vi "Init Plugin.vi"(8 "error in (no error)":errorcluster, 11 "RequestRestUI in":refnum<class "RequestRestUI.lvclass">) -> (0 "error out":errorcluster, 3 "RequestRestUI out":refnum<class "RequestRestUI.lvclass">)   [LabVIEW 2015]
uses:
  Plugin/Plugin.lvclass
  DatabaseManagement/Database.lvclass
  RequestRestUI.lvclass
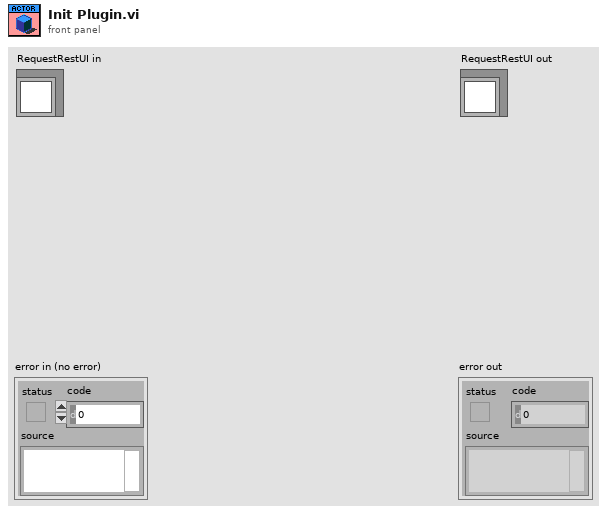
[diagram p1: front panel]
types:
  T1 = typedef "NI_Database_API.lvlib/DB Tools Column Info.ctl" = cluster{"column name":string, "data type":T2, "size":i32, "allow null?":bool}
  T2 = typedef "NI_Database_API.lvlib/DB Tools DataTypes.ctl" = enum16{"String", "Long (I32)", "Single (SGL)", "Double (DBL)", "Date/Time", "Binary"}
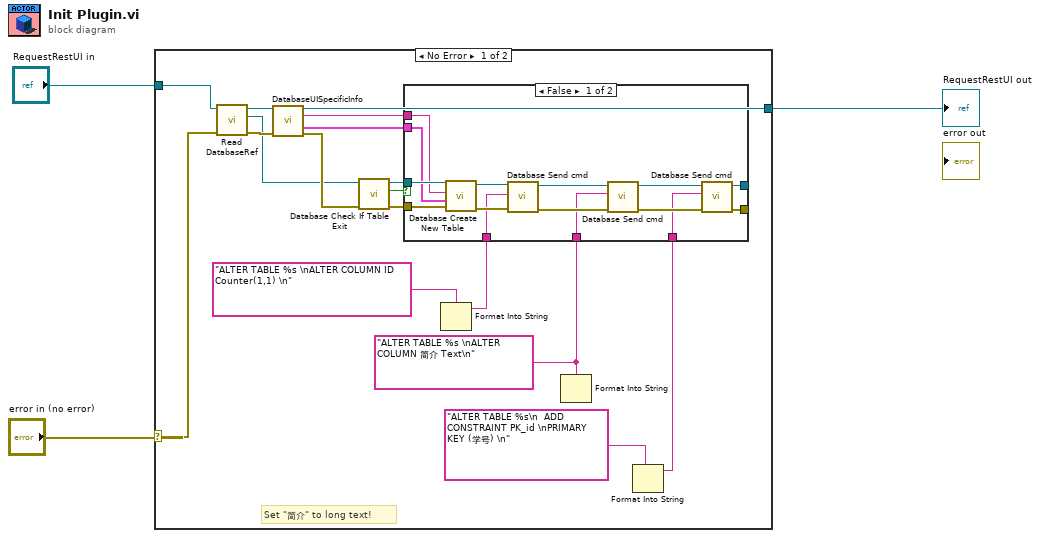
[diagram p0: block diagram]
diagram:
  n1 = case shown="No Error" "error in (no error)" {
    selector: "error in (no error)" -> [w11 _]
    tunnel: "RequestRestUI in" -> [w12 w38]
    tunnel: [w7 w38] -> w1
    frame No Error {
      w17 = "ALTER TABLE %s \nALTER COLUMN 简介 Text\n" ("SQL query")
      # "Set \"简介\" to long text!"
      n2 = call "Read DatabaseRef.vi"("error in (no error)"=w11, "Plugin in"=w12) -> ("error out"=w9:errorcluster, "Database.lvlib:Database"=w5:refnum<class "Database.lvclass">, "Plugin out"=w10:refnum<class "RequestRestUI.lvclass">)  [unwired: 7 in]
      n3 = call-dynamic "DatabaseUISpecificInfo.vi"("requestActor in"=w10, "error in (no error)"=w9) -> ("requestActor out"=w7:refnum<class "RequestRestUI.lvclass">, "TableName"=w8:string, "TableItemInfo"=w4:T1[], "error out"=w6:errorcluster)  [unwired: 9 in, 1 out]
      n4 = call "Database Check If Table Exit.vi"("error in (no error)"=w6, "Database in"=w5) -> ("error out"=w15:errorcluster, "Exit?"=w13:bool, "Database out"=w14:refnum<class "Database.lvclass">)  [unwired: 7 in]
      n5 = Format Into String(format string="ALTER TABLE %s \nALTER COLUMN ID Counter(1,1) \n" ("SQL query")) -> (resulting string=w19:string)  [unwired: 3 in, 1 out]
      n6 = Format Into String(format string=w17) -> ()  [unwired: 3 in, 2 out]
      n7 = Format Into String(format string="ALTER TABLE %s\n  ADD CONSTRAINT PK_id \nPRIMARY KEY (学号) \n" ("SQL query")) -> (resulting string=w20:string)  [unwired: 3 in, 1 out]
      n8 = case shown="False" w13 {
        tunnel: w14 -> [w35 w36]
        tunnel: w15 -> [w34 w37]
        tunnel: w8 -> [w33 _]
        tunnel: [w24 w37] -> _
        tunnel: [w25 w36] -> _
        tunnel: w17 -> [w28 _]
        tunnel: w19 -> [w23 _]
        tunnel: w20 -> [w22 _]
        tunnel: w4 -> [w21 _]
        frame False {
          n9 = call "Database Create New Table.vi"("error in (no error)"=w34, "column information"=w21, "table"=w33, "Database in"=w35) -> ("error out"=w31:errorcluster, "Database out"=w32:refnum<class "Database.lvclass">)  [unwired: 6 in]
          n10 = call "Database Send cmd.vi"("error in (no error)"=w31, "SQL query"=w23, "Database in"=w32) -> ("error out"=w29:errorcluster, "Database out"=w30:refnum<class "Database.lvclass">)  [unwired: 7 in]
          n11 = call "Database Send cmd.vi"("error in (no error)"=w29, "SQL query"=w28, "Database in"=w30) -> ("error out"=w26:errorcluster, "Database out"=w27:refnum<class "Database.lvclass">)  [unwired: 7 in]
          n12 = call "Database Send cmd.vi"("error in (no error)"=w26, "SQL query"=w22, "Database in"=w27) -> ("error out"=w24:errorcluster, "Database out"=w25:refnum<class "Database.lvclass">)  [unwired: 7 in]
        }
        frame True {
        }
      }
    }
    frame Error {
    }
  }
  "RequestRestUI out" <- w1
